vi "Monitor UA Flag.vi"(0 "OPC UA client refnum in":T2, 5 "NodeID In":string, 7 "Node SubArray In":string[](array[string]), 11 "error in (no error)":errorcluster) -> (4 "OPC UA client refnum out":T2, 6 "Subscription ID out":T1, 8 "NodeId Array Out":string[](array[string]), 10 "Event Registration Refnum Out":refnum<event-registration>, 15 "error out":errorcluster)   [LabVIEW 2024, in "OPCUA.lvlib"]
uses:
  <vilib>/OPCUA/controls/OPC UA Client Refnum.ctl
  <vilib>/OPCUA/controls/Subscription Data Change.ctl
  <vilib>/OPCUA/controls/NodeId.ctl
  <vilib>/OPCUA/controls/Data Type.ctl
  <vilib>/OPCUA/controls/OPC UA StatusCode.ctl
  <vilib>/OPCUA/controls/Subscription ID.ctl
  OPCUA.lvlib
  <vilib>/OPCUA/NI OPC UA Client.lvlib
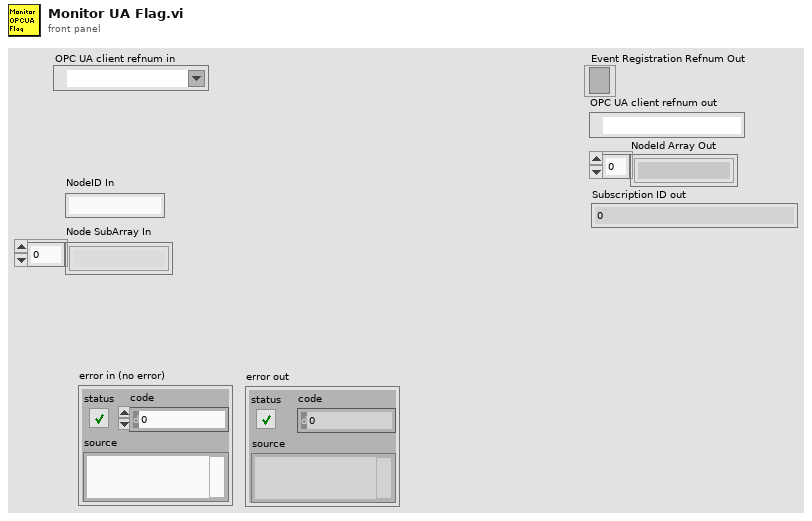
[diagram p1: front panel]
types:
  T1 = typedef "Subscription ID.ctl" = u32
  T2 = typedef "OPC UA Client Refnum.ctl" = refnum<k21>
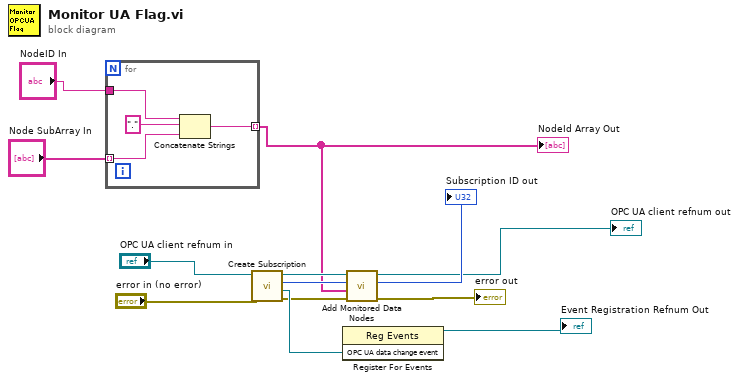
[diagram p0: block diagram]
diagram:
  n1 = for {
    tunnel: "Node SubArray In" -> [w14] mode=indexing
    tunnel: "NodeID In" -> [w15]
    tunnel: [w13] -> w1 mode=indexing
    n2 = Concatenate Strings(w15, ".", w14) -> (w13:string)
  }
  "NodeId Array Out" <- w1
  n3 = call <vilib>:"Create Subscription.vi"("error in (no error)"="error in (no error)", "OPC UA client refnum in"="OPC UA client refnum in") -> ("error out"=w8:errorcluster, "OPC UA data change event"=w10:refnum<user-event>, "subscription ID out"=w7:T1, "OPC UA client refnum out"=w9:T2)  [unwired: 5 in, 1 out]
  "Subscription ID out" <- w7
  n4 = register-events(w10) -> (reference out=→"Event Registration Refnum Out":refnum<event-registration>)  [unwired: 2 in, 1 out]
  n5 = call <vilib>:"Add Monitored Data Nodes.vi"("error in (no error)"=w8, "node IDs"=w1, "subscription ID in"=w7, "OPC UA client refnum in"=w9) -> ("error out"=→"error out":errorcluster, "OPC UA client refnum out"=→"OPC UA client refnum out":T2)  [unwired: 4 in, 2 out]
